vi "RankMinimalSchedule.vi"(8 "error in (no error)":errorcluster, 9 "Processing Time Matrix In":u16[][](array[numeric])=[[85, 23, 39, 55], [85, 74, 56, 78], [3, 96, 92, 11], [67, 45, 70, 75]], 10 "Number of Machines":i32=4, 11 "NUmber Of Jobs":i32=1) -> (0 "error out":errorcluster, 3 "Rank Minimal Matrix":i32[][](array[numeric]))   [LabVIEW 2013]
panel:
  out "Processing Time Matrix Out":i32[][](array[numeric])
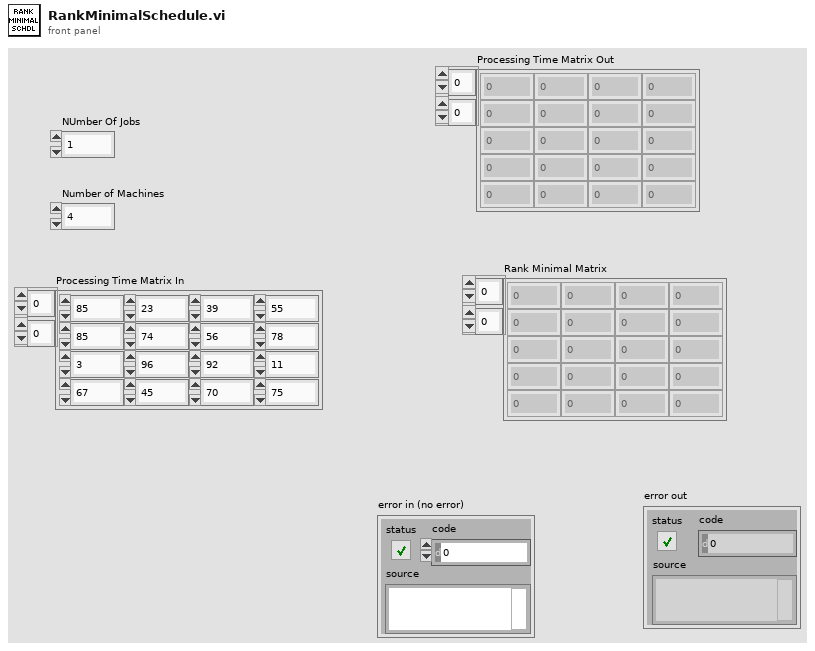
[diagram p1: front panel]
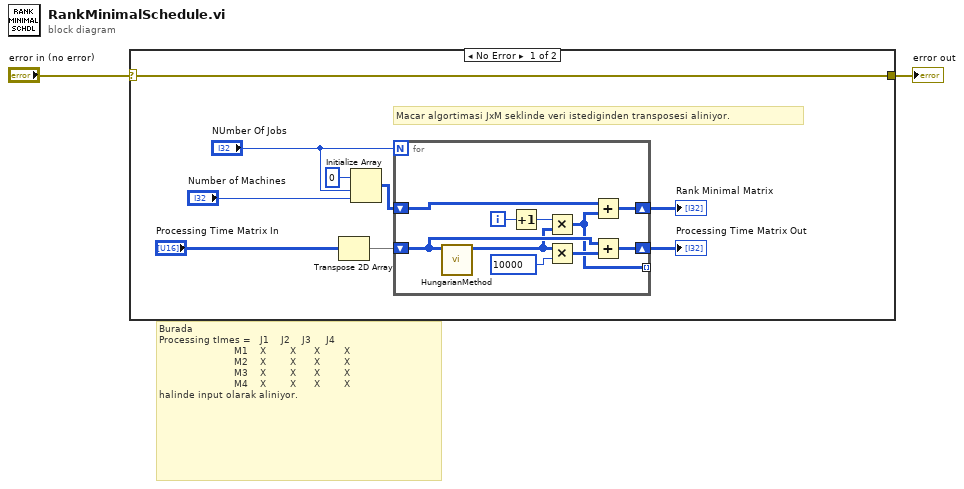
[diagram p0: block diagram]
diagram:
  # "Burada\nProcessing tImes =   J1    J2    J3     J4   \n                         M1    X        X      X        X\n                         M2    X        X      X        X\n                         M3    X        X      X        X\n                         M4    X        X      X        X\nhalinde input olarak aliniyor."
  n1 = case shown="No Error" "error in (no error)" {
    selector: "error in (no error)" -> [w5 w22]
    tunnel: [w5 w22] -> w1
    frame No Error {
      # "Macar algortimasi JxM seklinde veri istediginden transposesi aliniyor."
      n2 = Transpose 2D Array(2D array="Processing Time Matrix In") -> (transposed array=w3:u16[][])
      n3 = Initialize Array(0, "NUmber Of Jobs", "Number of Machines") -> (w8:i32[][])
      n4 = for {
        N: "NUmber Of Jobs" -> [_]
        shift-right: [w19] -> w11
        shift-left: w3 -> [w21]
        shift-right: [w13] -> w10
        shift-left: w8 -> [w14]
        tunnel: [w12] -> _ mode=indexing
        i -> [w17]
        n5 = call "HungarianMethod.vi"("Processing Time Matrix"=w21) -> ("Assignment"=w15:i8[][])  [unwired: 9 in, 1 out]
        n6 = Increment(x=w17) -> (x+1=w16:i32)
        n7 = Multiply(x=w16, y=w15) -> (x*y=w12:i32[][])
        n8 = Multiply(x=w15, y=10000) -> (x*y=w20:i32[][])
        n9 = Add(x=w14, y=w12) -> (x+y=w13:i32[][])
        n10 = Add(x=w21, y=w20) -> (x+y=w19:i32[][])
      }
      "Processing Time Matrix Out" <- w11
      "Rank Minimal Matrix" <- w10
    }
    frame Error {
    }
  }
  "error out" <- w1
